vi "Front Panel Controls.vi"(8 "error in (no error)":errorcluster, 11 "VI/Type-Def Path":path) -> (0 "error out":errorcluster, 3 "Controls[]":refnum<vi>[](array[refnum]))   [LabVIEW 2018, in "Scripting.lvlib"]
uses:
  Scripting.lvlib
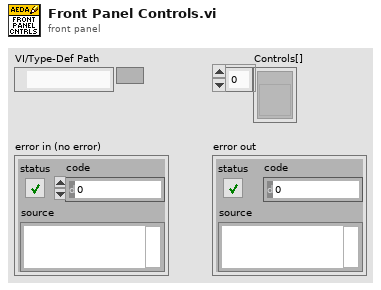
[diagram p1: front panel]
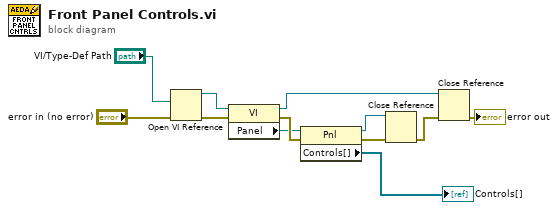
[diagram p0: block diagram]
diagram:
  n1 = Open VI Reference(vi path="VI/Type-Def Path", error in (no error)="error in (no error)") -> (vi reference=w4:refnum<vi>, error out=w3:errorcluster)  [unwired: 4 in]
  n2 = property class="VI"(reference=w4, error in=w3) -> (reference out=w6:refnum<vi>, error out=w11:errorcluster, "Panel"=w5:refnum<vi>)
  n3 = property class="Pnl"(reference=w5, error in=w11) -> (reference out=w7:refnum<vi>, error out=w8:errorcluster, "Controls[]"=→"Controls[]":refnum<vi>[])
  n4 = Close Reference(reference=w7, error in (no error)=w8) -> (error out=w9:errorcluster)
  n5 = Close Reference(reference=w6, error in (no error)=w9) -> (error out=→"error out":errorcluster)
